vi "SmartSEM Remote API FIB gun state.vi"(8 "error in":errorcluster, 11 "ActiveX Container":refnum<k7>(container)) -> (0 "error out":errorcluster={"status"=FALSE, "code"=-2147417851, "source"=""}, 2 "FIB Gun State":string, 3 "reference out":refnum<k7>)   [LabVIEW 2018]
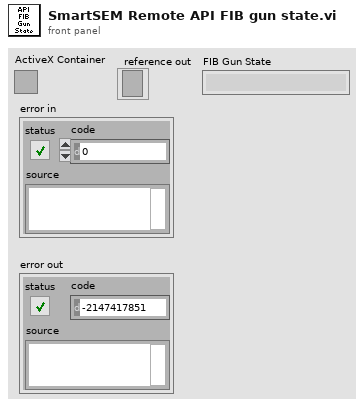
[diagram p1: front panel]
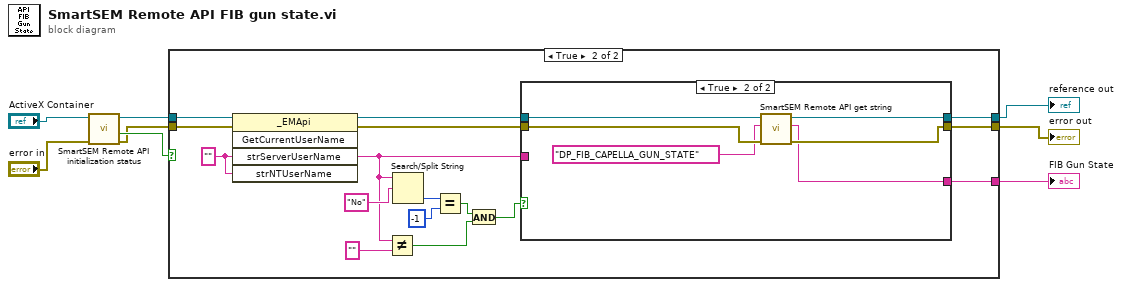
[diagram p0: block diagram]
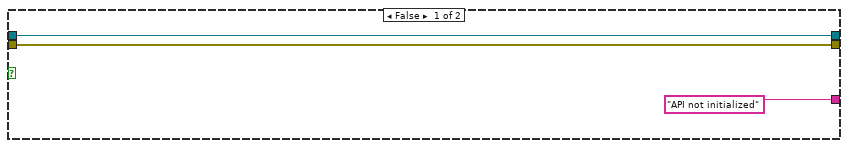
[diagram p2: hidden frame]
diagram:
  n1 = call "SmartSEM Remote API initialization status.vi"("error in"="error in", "ActiveX Container"="ActiveX Container") -> ("error out"=w4:errorcluster, "API initialized"=w5:bool, "reference out"=w3:refnum<k7>)  [unwired: 7 in]
  n2 = case shown="True" w5 {
    tunnel: w3 -> [w10 w18]
    tunnel: w4 -> [w9 w17]
    tunnel: [w10 w27] -> w1
    tunnel: [w9 w26] -> w8
    tunnel: ["API not initialized" ("lpszParam") w22] -> w7
    frame False {
    }
    frame True {
      w23 = "" ("strServerUserName")
      n3 = invoke class="_EMApi" method="GetCurrentUserName"(reference=w18, error in=w17, "strServerUserName"=w23, "strNTUserName"=w23) -> (reference out=w25:refnum<k7>, error out=w24:errorcluster, "strServerUserName"=w16:string)  [unwired: 1 in, 2 out]
      n4 = Not Equal?(x=w16, y="") -> (x != y?=w12:bool)
      n5 = Search/Split String(string=w16, search string/char (-)="No" ("strServerUserName")) -> (offset of match=w20:i32)  [unwired: 1 in, 2 out]
      n6 = Equal?(x=w20, y=-1) -> (x = y?=w14:bool)
      n7 = And(x=w14, y=w12) -> (x .and. y?=w13:bool)
      n8 = case shown="True" w13 {
        tunnel: [w30 w33] -> w27
        tunnel: [w29 w32] -> w26
        tunnel: w25 -> [w30 w36]
        tunnel: w24 -> [w29 w35]
        tunnel: [w28 w31] -> w22
        tunnel: w16 -> [w28 _]
        frame False {
        }
        frame True {
          n9 = call "SmartSEM Remote API get string.vi"("error in"=w35, "lpszParam"="DP_FIB_CAPELLA_GUN_STATE", "ActiveX Container"=w36) -> ("error out"=w32:errorcluster, "data"=w31:string, "reference out"=w33:refnum<k7>)  [unwired: 6 in]
        }
      }
    }
  }
  "error out" <- w8
  "FIB Gun State" <- w7
  "reference out" <- w1
